vi "place_of_mark.vi"(11 "pieceOfWorld in":T1[][](array[typedef])) -> (3 "f":i32)   [LabVIEW 2015, in "PolyVIEW.lvclass"]
uses:
  PolyVIEW.lvclass
  actors/world/typedefs/worldCell_cluster.ctl
  actors/world/typedefs/markValue_cluster.ctl
  actors/world/typedefs/markValue.ctl
  actors/world/typedefs/markVolume.ctl
  actors/world/typedefs/amountOfFood.ctl
  actors/world/typedefs/anthillType_enum.ctl
  actors/world/world.lvlib
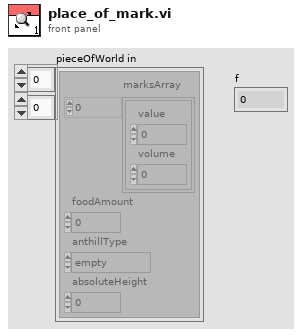
[diagram p1: front panel]
types:
  T1 = typedef "world.lvlib/worldCell_cluster.ctl" = cluster{"marksArray":T2[], "foodAmount":T5, "anthillType":T6, "absoluteHeight":u8}
  T2 = typedef "world.lvlib/markValue_cluster.ctl" = cluster{"value":T3, "volume":T4}
  T3 = typedef "world.lvlib/markValue.ctl" = u8
  T4 = typedef "world.lvlib/markVolume.ctl" = u16
  T5 = typedef "world.lvlib/amountOfFood.ctl" = i32
  T6 = typedef "world.lvlib/anthillType_enum.ctl" = enum16{"empty", "own", "rival"}
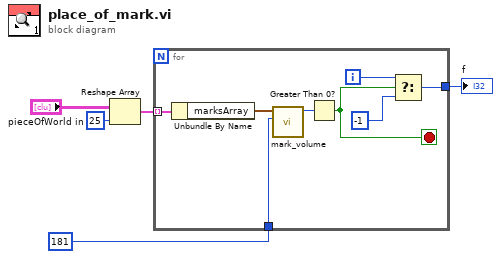
[diagram p0: block diagram]
diagram:
  n1 = Reshape Array("pieceOfWorld in", 25 ("dimension size")) -> (w2:T1[])
  n2 = for {
    tunnel: w2 -> [w13] mode=indexing
    tunnel: [w8] -> w5
    tunnel: T3 181 ("element") -> [w7]
    i -> [w9]
    stop <- w10 stop-if-true
    n3 = Unbundle By Name(w13) -> ("marksArray"=w12:T2[])
    n4 = call "mark_volume.vi"("element"=w7, "marksArray"=w12) -> ("volume"=w11:T4)  [unwired: 9 in]
    n5 = Greater Than 0?(x=w11) -> (x > 0?=w10:bool)
    n6 = Select(t=w9, s=w10, f=-1) -> (s? t:f=w8:i32)
  }
  "f" <- w5
